vi "Log Data.vi"(8 "error in (no error)":errorcluster, 10 "Data Queue":refnum<queue>, 11 "Logging Configuration":T1) -> (0 "error out":errorcluster)   [LabVIEW 2018, in "Logging.lvlib"]
doc: "This VI uses the TDMS Write function to write data to a TDMS file."
uses:
  Logging.lvlib
  Logging Configuration.ctl
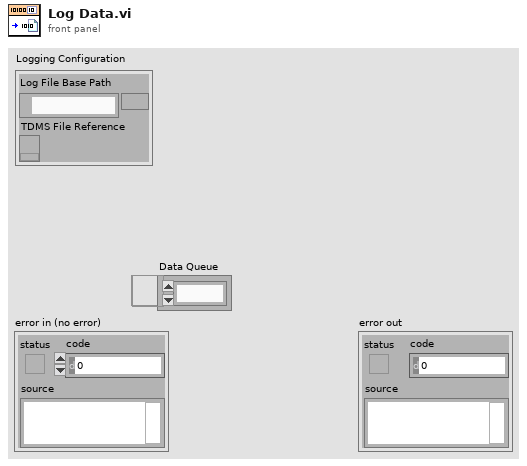
[diagram p1: front panel]
types:
  T1 = typedef "Logging.lvlib/Logging Configuration.ctl" = cluster{"Log File Base Path":path, "TDMS File Reference":refnum<k34>}
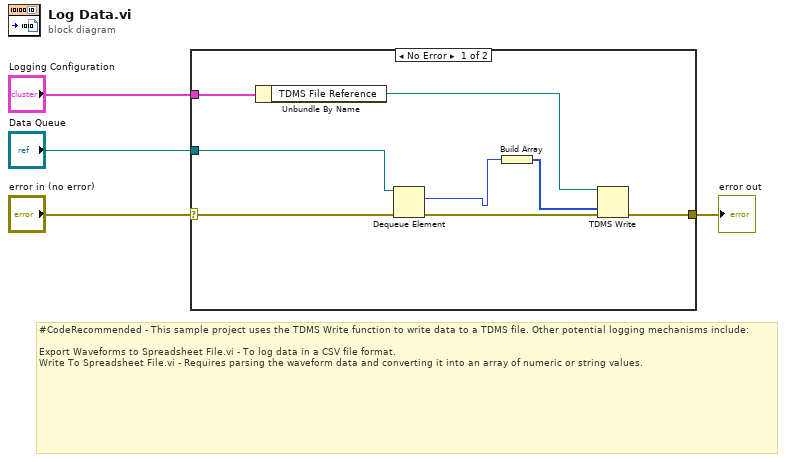
[diagram p0: block diagram]
diagram:
  # "#CodeRecommended - This sample project uses the TDMS Write function to write data to a TDMS file. Other potential logging mechanisms include:\n\nExport Waveforms to Spreadsheet File.vi - To log data in a CSV file format.\nWrite To Spreadsheet File.vi - Requires parsing the waveform data and converting it into an array of numeric or string values."
  n1 = case shown="No Error" "error in (no error)" {
    selector: "error in (no error)" -> [w10 w13]
    tunnel: "Logging Configuration" -> [w12 _]
    tunnel: "Data Queue" -> [w9 _]
    tunnel: [w11 w13] -> w2
    frame No Error {
      n2 = Unbundle By Name(w12) -> ("TDMS File Reference"=w7:refnum<k34>)
      n3 = Dequeue Element(queue=w9, error in (no error)=w10) -> (element=w6:u32, error out=w8:errorcluster)  [unwired: 1 in, 2 out]
      n4 = Build Array(w6) -> (w5:u32[])
      n5 = TDMS Write(0:w7, 9:w5, 11:w8) -> (15:w11:errorcluster)  [unwired: 3 in, 3 out]
    }
    frame Error {
    }
  }
  "error out" <- w2
